vi "Add secondaries coincidence flag.vi"(1 "Hits in":u64[](array[numeric])) -> (0 "Array":T1(array[cluster]))   [LabVIEW 2016]
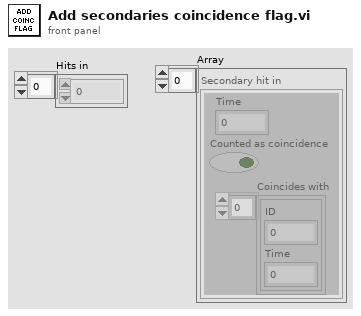
[diagram p1: front panel]
types:
  T1 = cluster{"Time":u64, "Counted as coincidence":bool, "Coincides with":cluster{"ID":i8, "Time":u64}[]}[]
  T2 = cluster{"Time":u64, "Counted as coincidence":bool, "Coincides with":cluster{"ID":i8, "Time":u64}[]}
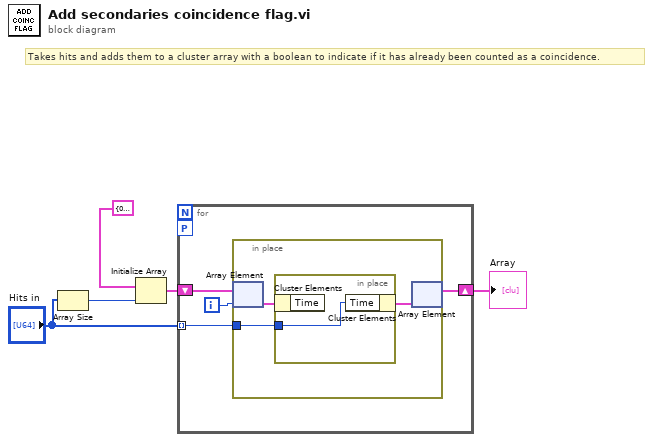
[diagram p0: block diagram]
diagram:
  # "Takes hits and adds them to a cluster array with a boolean to indicate if it has already been counted as a coincidence."
  n1 = Array Size(array="Hits in") -> (size(s)=w4:i32)
  n2 = Initialize Array(T2 {"Time"=0, "Counted as coincidence"=FALSE, "Coincides with"=[]} ("Secondary hit in"), w4) -> (w5:T1)
  n3 = for {
    tunnel: "Hits in" -> [w7] mode=indexing
    shift-right: [w6] -> w2
    shift-left: w5 -> [w9]
    workers-P: _ -> [_]
    i -> [w8]
    n4 = in-place {
      in-place-border: w7 -> [w11]
      n5 = in-place-array #1(w9, w8) -> (w12:T2)
      n6 = in-place {
        in-place-border: w11 -> [w13]
        n7 = in-place-cluster #2(w12) -> ()  [unwired: 1 out]
        n8 = in-place-cluster #2("Time"=w13) -> (w10:T2)
      }
      n9 = in-place-array #1(w10) -> (w6:T1)  [unwired: 1 out]
    }
  }
  "Array" <- w2
